vi "testReadXMLTime.vi"() -> ()   [LabVIEW 2009, in "run.lvlib"]
uses:
  Hal/testing/run.lvlib
  PixelflySettings.lvclass
  Filing/FileSystem/FileSystem.lvclass
  CamaraSettings.lvclass
panel:
  in  "stop":bool=TRUE
  out "exposure_time":dbl
  out "total":dbl format="%_6g"
  out "load":dbl format="%_6g"
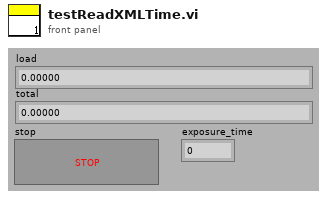
[diagram p1: front panel]
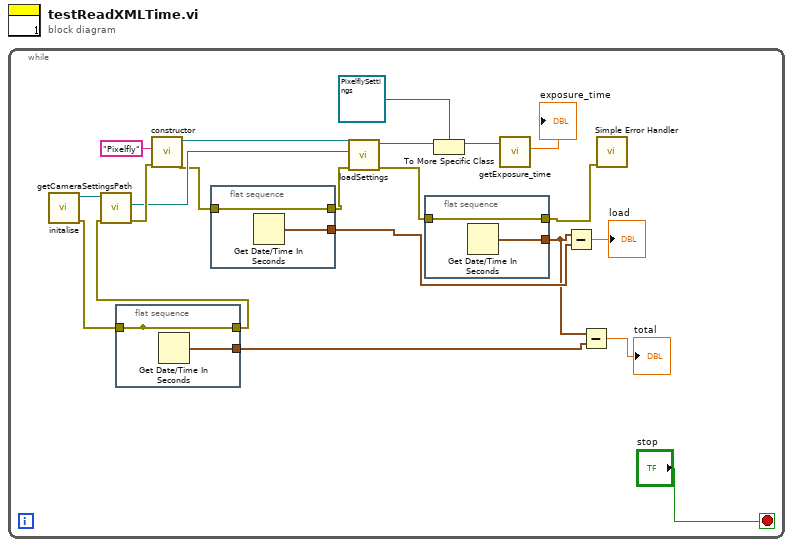
[diagram p0: block diagram]
diagram:
  n1 = while {
    stop <- "stop" stop-if-true
    n2 = call "initalise.vi"() -> ("error out"=w12:errorcluster, "FileSystem out"=w19:refnum<class "FileSystem.lvclass">)  [unwired: 10 in]
    n3 = call-dynamic "getCameraSettingsPath.vi"("error in (no error)"=w11, "FileSystem.lvclass in"=w19) -> ("error out"=w18:errorcluster, "CameraSettingsPath"=w17:path)  [unwired: 7 in, 1 out]
    n4 = flat-sequence {
      tunnel: [w22] -> _
      tunnel: [w22] -> w11
      tunnel: [w23] -> w9
      tunnel: w12 -> [w22]
      frame #0 {
        n5 = Get Date/Time In Seconds() -> (seconds since 1Jan1904=w23:timestamp)
      }
    }
    n6 = call "constructor.vi"("error in (no error)"=w18, "camera settings"="Pixelfly") -> ("error out"=w16:errorcluster, "CamaraSettings out"=w20:refnum<class "CamaraSettings.lvclass">)  [unwired: 8 in]
    n7 = flat-sequence {
      tunnel: w16 -> [w27]
      tunnel: [w27] -> w15
      tunnel: [w26] -> w14
      frame #0 {
        n8 = Get Date/Time In Seconds() -> (seconds since 1Jan1904=w26:timestamp)
      }
    }
    n9 = call-dynamic "loadSettings.vi"("error in (no error)"=w15, "Path"=w17, "CamaraSettings in"=w20) -> ("error out"=w3:errorcluster, "CamaraSettings out"=w6:refnum<class "CamaraSettings.lvclass">)  [unwired: 7 in]
    n10 = flat-sequence {
      tunnel: w3 -> [w25]
      tunnel: [w25] -> w7
      tunnel: [w24] -> w10
      frame #0 {
        n11 = Get Date/Time In Seconds() -> (seconds since 1Jan1904=w24:timestamp)
      }
    }
    n12 = To More Specific Class(target class=refnum<class "PixelflySettings.lvclass"> refnum ("Tools.lvlib:Settings.lvlib:PixelflySettings.lvclass"), reference=w6) -> (specific class reference=w5:refnum<class "PixelflySettings.lvclass">)  [unwired: 1 in, 1 out]
    n13 = call "getExposure_time.vi"("PixelflySettings in"=w5) -> ("exposure_time"=→"exposure_time":dbl)  [unwired: 8 in, 2 out]
    n14 = Subtract(x=w10, y=w14) -> (x-y=→"load":dbl)
    n15 = Subtract(x=w10, y=w9) -> (x-y=→"total":dbl)
    n16 = call <vilib>:"Simple Error Handler.vi"("error in (no error)"=w7) -> ()  [unwired: 4 in, 5 out]
  }
